vi "Robot Main.vi"() -> ()   [LabVIEW 2012]
doc: "This VI imlements the framework and scheduler for your robotics program. It should not be necessary to modify the framework. You are expected to add your code to the VIs called from Robot Main, the ones located in the Team Code within the project."
uses:
  <vilib>/Rock Robotics/WPI/Camera/WPI_CameraImageSize.ctl
  Robot Global Data.vi
panel:
  in  "Image Size":T1=enum."320x240"
  in  "Enable Vision":bool
  in  "Finish":bool
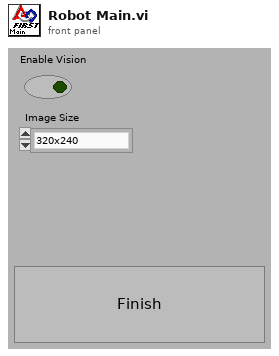
[diagram p1: front panel]
types:
  T1 = typedef "WPI_CameraImageSize.ctl" = enum16{"640x480", "320x240", "160x120"}
  T2 = typedef "WPI_DriverStationMatch Info.ctl" = cluster{"Autonomous Elapsed Seconds":dbl, "TeleOp Elapsed Seconds":dbl, "Disabled Elapsed Seconds":dbl, "Visited Autonomous":bool, "Visited TeleOp":bool, "Visited Disabled":bool, "Autonomous Settings":cluster{"Autonomous Style":enum16{"Iterative", "Independent"}, "VI Refnum":refnum<vi>}}
  T3 = typedef "WPI_DriverStationDerivedRobotMode.ctl" = enum16{"Init", "Execute", "Stop"}
  T4 = typedef "WPI_DriverStationRobotMode2.ctl" = enum16{"Autonomous Disabled", "Autonomous Enabled", "Teleop Disabled", "Teleop Enabled", "Timeout", "Finish", "Test Disabled", "Test Enabled"}
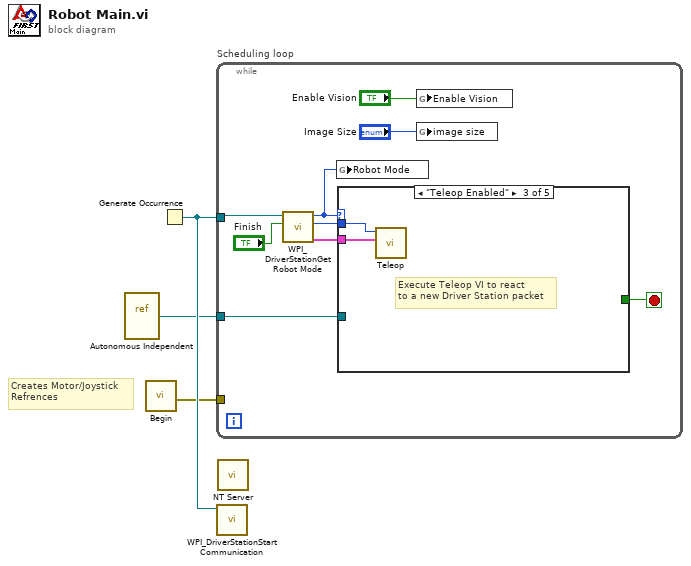
[diagram p0: block diagram]
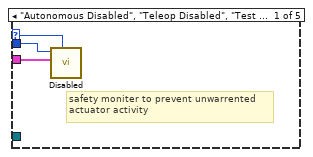
[diagram p2: hidden frame]
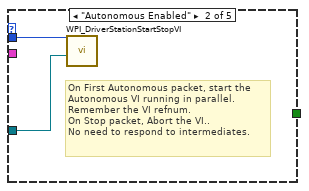
[diagram p3: hidden frame]
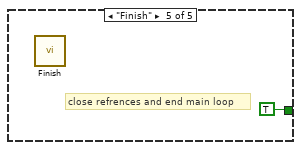
[diagram p5: hidden frame]
diagram:
  # "Creates Motor/Joystick\nRefrences"
  n1 = vi-ref "Autonomous Independent.vi"() -> (w2:refnum<vi>)
  n2 = call "Begin.vi"() -> ("error constant"=w1:errorcluster)  [unwired: 1 in, 10 out]
  n3 = Generate Occurrence() -> (w3:refnum<k4>)
  n4 = while "Scheduling loop" {
    tunnel: w3 -> [w11]
    tunnel: w1 -> [_]
    tunnel: w2 -> [w6]
    stop <- w8 stop-if-true
    n5 = call <vilib>:"WPI_DriverStationGet Robot Mode.vi"("Finish"="Finish", "DS Occurrence"=w11) -> ("Match Info out"=w9:T2, "Call Context"=w12:T3, "Robot Mode"=w4:T4)  [unwired: 7 out]
    n6 = global write "Robot Global Data.vi" "Robot Mode"(w4) -> ()
    n7 = case shown="\"Teleop Enabled\"" w4 {
      selector: w4 -> [w13 _ _ _ _]
      tunnel: w12 -> [w15 w17 w19 _ _]
      tunnel: w9 -> [w14 _ w18 _ _]
      tunnel: [_ _ _ _ TRUE] -> w8
      tunnel: w6 -> [_ w16 _ _ _]
      frame "Autonomous Disabled", "Teleop Disabled", "Test Disabled", "Test Enabled" {
        # "safety moniter to prevent unwarrented\nactuator activity"
        n8 = call "Disabled.vi"("Robot Mode"=w13, "Match Info"=w14, "Call Context"=w15) -> ()  [unwired: 1 in, 8 out]
      }
      frame "Autonomous Enabled" {
        # "On First Autonomous packet, start the\nAutonomous VI running in parallel.\nRemember the VI refnum.\nOn Stop packet, Abort the VI..\nNo need to respond to intermediates."
        n9 = call <vilib>:"WPI_DriverStationStartStopVI.vi"("VI in"=w16, "Call Context"=w17) -> ()  [unwired: 10 in]
      }
      frame "Teleop Enabled" {
        # "Execute Teleop VI to react\nto a new Driver Station packet"
        n10 = call "Teleop.vi"("Match Info"=w18, "Call Context"=w19) -> ()  [unwired: 1 in, 9 out]
      }
      frame "Timeout" {
        # "Driver Station packet didn't arrive.\nPossibly useful for diagnostics"
      }
      frame "Finish" {
        # "close refrences and end main loop"
        n11 = call "Finish.vi"() -> ()  [unwired: 1 in, 7 out]
      }
    }
    n12 = global write "Robot Global Data.vi" "Enable Vision"("Enable Vision") -> ()
    n13 = global write "Robot Global Data.vi" "image size"("Image Size") -> ()
  }
  n14 = call <vilib>:"WPI_DriverStationStart Communication.vi"("occurrence"=w3) -> ()  [unwired: 11 out]
  n15 = call <vilib>:"NT Server.vi"() -> ()  [unwired: 12 in]
